vi "test_AlarmColors.vi"() -> ()   [LabVIEW 2009]
uses:
  controls/sec_AlarmStatus_cluster.ctl
  modules/alarm colors/sec_AlarmColors_Command_enum.ctl
  controls/sec_AlarmStates_enum.ctl
panel:
  out "Zone Status Indicators":T1
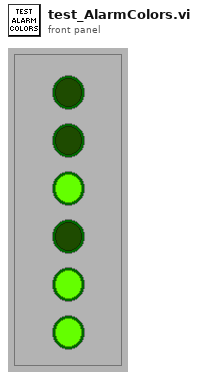
[diagram p1: front panel]
types:
  T1 = typedef "sec_AlarmStatus_cluster.ctl" = cluster{"Boolean":bool, "Boolean 2":bool, "Boolean 3":bool, "Boolean 4":bool, "Boolean 5":bool, "Boolean 6":bool}
  T2 = typedef "sec_AlarmStates_enum.ctl" = enum16{"Normal", "Alarm", "Bypass", "Tamper"}
  T3 = typedef "sec_AlarmColors_Command_enum.ctl" = enum16{"Initialise", "Set Alarm States", "Update Alarm Status Display", "Shutdown"}
  T4 = cluster{"Alarm Status[0]":bool, "Alarm Status[1]":bool, "Alarm Status[2]":bool, "Alarm Status[3]":bool, "Alarm Status[4]":bool, "Alarm Status[5]":bool}
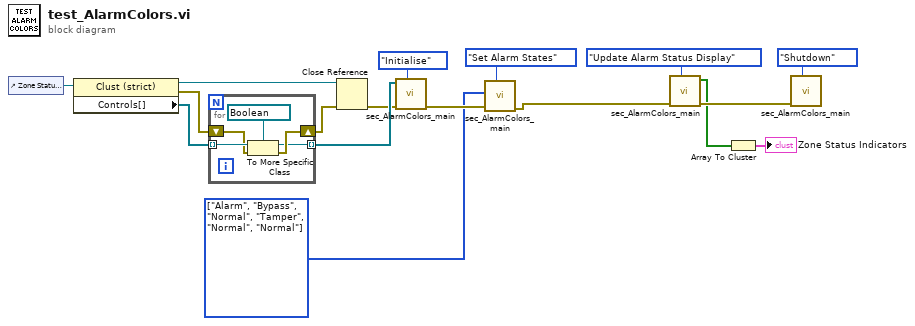
[diagram p0: block diagram]
diagram:
  w4 = T2[] [enum."Alarm", enum."Bypass", enum."Normal", enum."Tamper", enum."Normal", enum."Normal"] items=["Normal", "Alarm", "Bypass", "Tamper"] ("Alarm States")
  n1 = control-ref of="Zone Status Indicators"() -> (w10:refnum<vi>)
  n2 = property class="Clust (strict)"(reference=w10) -> (reference out=w6:refnum<vi>, error out=w8:errorcluster, "Controls[]"=w9:refnum<vi>[])  [unwired: 1 in]
  n3 = for {
    tunnel: w9 -> [w22] mode=indexing
    shift-right: [w20] -> w7
    shift-left: w8 -> [w21]
    tunnel: [w18] -> w5 mode=indexing
    n4 = To More Specific Class(target class=refnum<vi> refnum ("specific class reference"), reference=w22, error in=w21) -> (specific class reference=w18:refnum<vi>, error out=w20:errorcluster)
  }
  n5 = Close Reference(reference=w6, error in (no error)=w7) -> (error out=w1:errorcluster)
  n6 = call "sec_AlarmColors_main.vi"("Command"=sec_AlarmColors_Command_enum."Initialise", "error in (no error)"=w1, "Status Zone Refnums"=w5) -> ("error out"=w13:errorcluster)  [unwired: 7 in, 1 out]
  n7 = call "sec_AlarmColors_main.vi"("Command"=sec_AlarmColors_Command_enum."Set Alarm States", "error in (no error)"=w13, "Alarm States"=w4) -> ("error out"=w12:errorcluster)  [unwired: 7 in, 1 out]
  n8 = call "sec_AlarmColors_main.vi"("Command"=sec_AlarmColors_Command_enum."Update Alarm Status Display", "error in (no error)"=w12) -> ("error out"=w11:errorcluster, "Alarm Status"=w3:bool[])  [unwired: 8 in]
  n9 = Array To Cluster(array=w3) -> (cluster=→"Zone Status Indicators":T4)
  n10 = call "sec_AlarmColors_main.vi"("Command"=sec_AlarmColors_Command_enum."Shutdown", "error in (no error)"=w11) -> ()  [unwired: 8 in, 2 out]
